vi "Startup_proximity.vi"(6 "LabVIEW Web Service":refnum<class "Web Service.lvclass">) -> ()   [LabVIEW 2019]
uses:
  <vilib>/wsapi/Web Service.lvclass
  <vilib>/httpClient/POSTBuffer.vi
  <vilib>/httpClient/LabVIEWHTTPClient.lvlib
panel:
  out "Publish Response":string[](array[string])
  # "Use the web service input terminal to call the VIs on the Service subpalette of the Web Services palette. Do not remove it from the connector pane unless you don't need access to the palette."
  # "Any additional terminals added to the connector pane of a startup VI will be ignored."
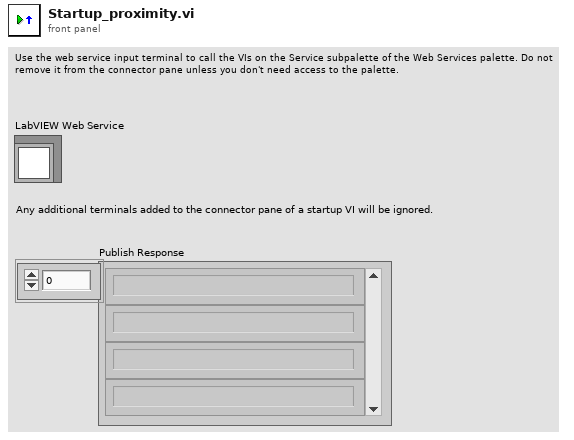
[diagram p1: front panel]
types:
  T1 = cluster{"name":string, "value":dbl[], "source":string}
  T2 = cluster{"name":string, "value":dbl[], "source":string}[]
  T3 = typedef "LabVIEWHTTPClient.lvlib/ClientHandle.ctl" = refnum<k1>
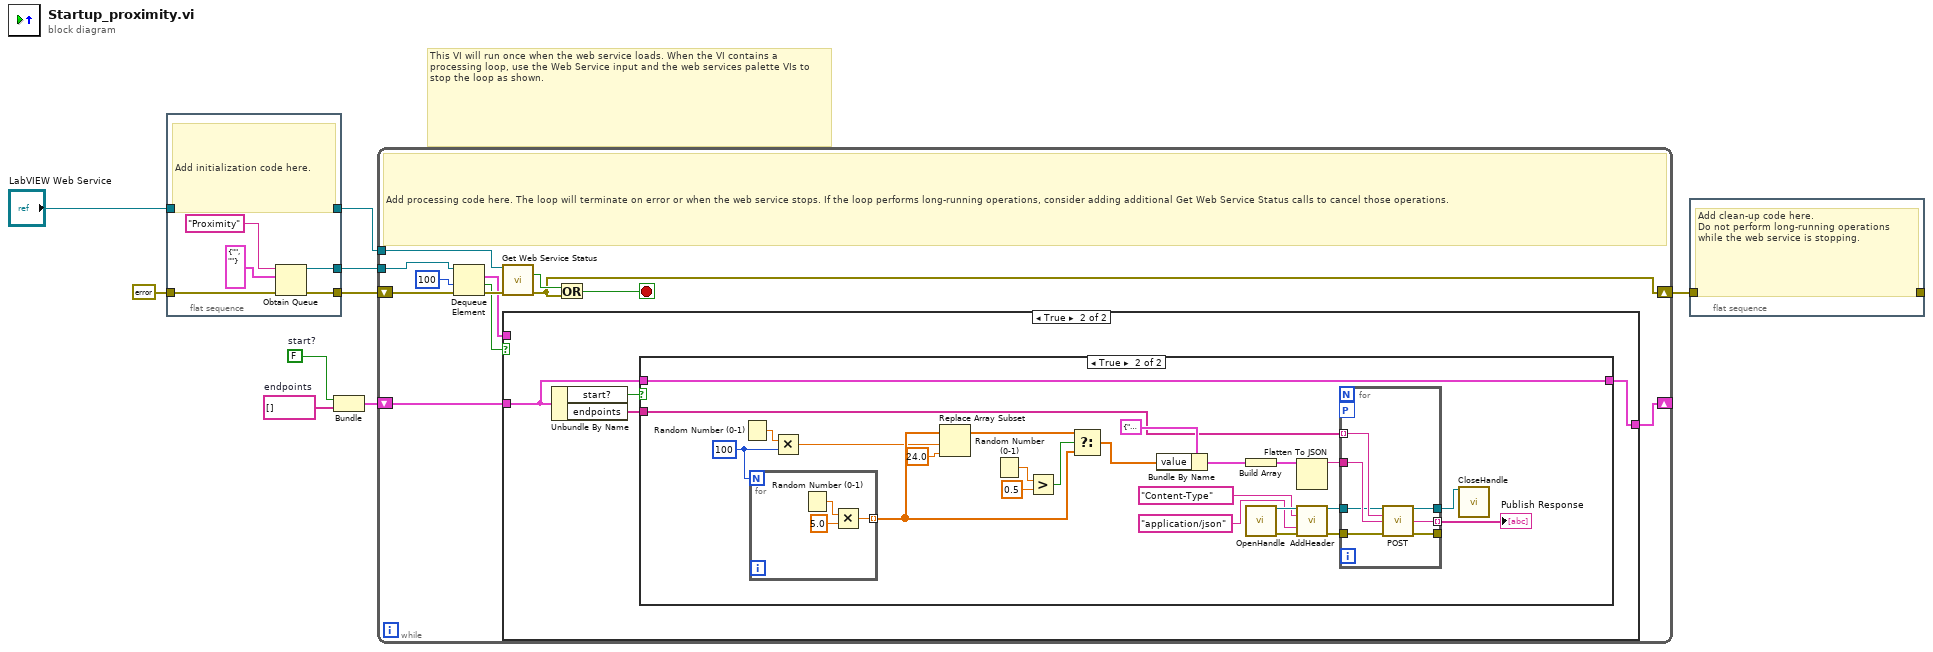
[diagram p0: block diagram]
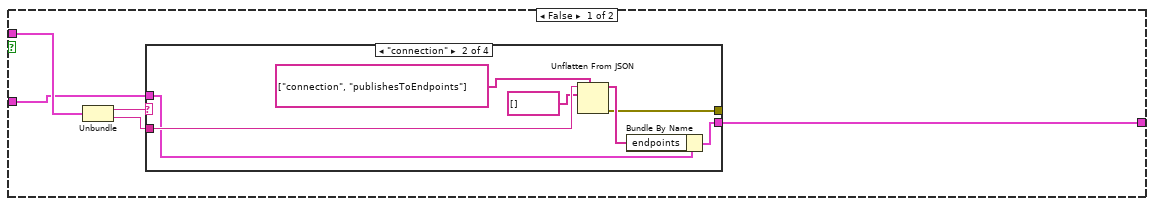
[diagram p2: hidden frame]
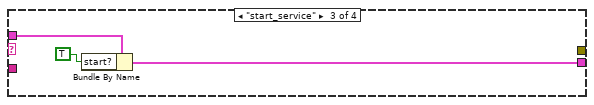
[diagram p4: hidden frame]
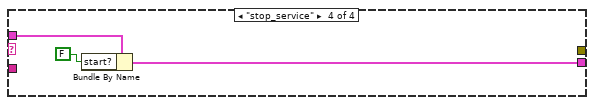
[diagram p5: hidden frame]
diagram:
  w1 = string[] []  # endpoints
  w3 = FALSE  # start?
  # "This VI will run once when the web service loads. When the VI contains a processing loop, use the Web Service input and the web services palette VIs to stop the loop as shown."
  n1 = flat-sequence {
    tunnel: "LabVIEW Web Service" -> [w15]
    tunnel: [w15] -> w8
    tunnel: [w11] -> w7
    tunnel: errorcluster {"status"=FALSE, "code"=0, "source"=""} ("error constant") -> [w10]
    tunnel: [w12] -> w4
    frame #0 {
      # "Add initialization code here."
      n2 = Obtain Queue(name (unnamed)="Proximity", element data type=cluster{string, "postdata":string} {"", "postdata"=""} ("output cluster"), error in (no error)=w10) -> (queue out=w12:refnum<queue>, error out=w11:errorcluster)  [unwired: 2 in, 1 out]
    }
  }
  n3 = Bundle("start?"=w3, "endpoints"=w1) -> (w2:cluster{"start?":bool, "endpoints":string[]})  [unwired: 1 in]
  n4 = while {
    tunnel: w8 -> [w26]
    shift-right: [w24] -> w5
    shift-left: w7 -> [w23]
    tunnel: w4 -> [w21]
    shift-right: [w16] -> _
    shift-left: w2 -> [w18]
    stop <- w25 stop-if-true
    # "Add processing code here. The loop will terminate on error or when the web service stops. If the loop performs long-running operations, consider adding additional Get Web Service Status calls to cancel those operations."
    n5 = Dequeue Element(queue=w21, timeout in ms (-1)=100, error in (no error)=w23) -> (element=w17:cluster{string, "postdata":string}, timed out?=w19:bool, error out=w22:errorcluster)  [unwired: 1 out]
    n6 = call <vilib>:"Get Web Service Status.vi"("LabVIEW Web Service"=w26, "error in (no error)"=w22) -> ("service stopping?"=w27:bool, "error out"=w24:errorcluster)  [unwired: 11 in, 1 out]
    n7 = case shown="True" w19 {
      tunnel: w18 -> [w29 w48]
      tunnel: w17 -> [w32 _]
      tunnel: [w28 w49] -> w16
      frame False {
        n8 = Unbundle(w32) -> (w31:string, "postdata"=w30:string)
        n9 = case shown="\"connection\"" w31 {
          tunnel: w30 -> [_ w40 _ _]
          tunnel: w29 -> [w33 w37 w43 w46]
          tunnel: [_ w35 _ _] -> _
          tunnel: [w33 w34 w42 w45] -> w28
          frame Default {
          }
          frame "connection" {
            n10 = Unflatten From JSON(path=string[] ["connection", "publishesToEndpoints"], JSON string=w40, type and defaults=string[] [] ("path")) -> (value=w36:string[], error out=w35:errorcluster)  [unwired: 4 in]
            n11 = Bundle By Name(cluster=w37, "endpoints"=w36) -> (w34:cluster{"start?":bool, "endpoints":string[]})
          }
          frame "start_service" {
            n12 = Bundle By Name(cluster=w43, "start?"=TRUE) -> (w42:cluster{"start?":bool, "endpoints":string[]})
          }
          frame "stop_service" {
            n13 = Bundle By Name(cluster=w46, "start?"=FALSE) -> (w45:cluster{"start?":bool, "endpoints":string[]})
          }
        }
      }
      frame True {
        n14 = Unbundle By Name(w48) -> ("start?"=w50:bool, "endpoints"=w47:string[])
        n15 = case shown="True" w50 {
          tunnel: [w51 w75] -> w49
          tunnel: w48 -> [w51 w75]
          tunnel: w47 -> [_ w63]
          frame False {
          }
          frame True {
            w66 = 100
            n16 = Random Number (0-1)() -> (number: 0 to 1=w67:dbl)
            n17 = for {
              N: w66 -> [_]
              tunnel: [w83] -> w70 mode=indexing
              n18 = Random Number (0-1)() -> (number: 0 to 1=w85:dbl)
              n19 = Multiply(x=w85, y=5.0) -> (x*y=w83:dbl)
            }
            n20 = Multiply(x=w67, y=w66) -> (x*y=w65:dbl)
            n21 = Replace Array Subset(array=w70, new element=24.0 ("new element/subarray"), index=w65) -> (w69:dbl[])
            n22 = Random Number (0-1)() -> (number: 0 to 1=w73:dbl)
            n23 = Greater?(x=w73, y=0.5) -> (0:w72:bool)
            n24 = Select(t=w69, s=w72, f=w70) -> (s? t:f=w71:dbl[])
            n25 = Bundle By Name(cluster=T1 {"name"="Promximity Sensor", "value"=[], "source"="Promximity Sensor"}, "value"=w71) -> (w62:T1)
            n26 = Build Array(w62) -> (w61:T2)
            n27 = call <vilib>:"OpenHandle.vi"() -> ("client handle out"=w57:T3, "error out"=w56:errorcluster)  [unwired: 14 in]
            n28 = Flatten To JSON(anything=w61) -> (JSON string=w60:string)  [unwired: 2 in, 1 out]
            n29 = call <vilib>:"AddHeader.vi"("client handle"=w57, "header"="Content-Type", "value"="application/json", "error in (no error)"=w56) -> ("client handle out"=w54:T3, "error out"=w55:errorcluster)  [unwired: 10 in]
            n30 = for {
              tunnel: w63 -> [w82] mode=indexing
              tunnel: w60 -> [w81]
              tunnel: [w80] -> w59 mode=indexing
              workers-P: _ -> [_]
              tunnel: w55 -> [w77]
              tunnel: [w76] -> _
              tunnel: w54 -> [w79]
              tunnel: [w78] -> w58
              n31 = call-poly <vilib>:"POST.vi"("client handle"=w79, "url"=w82, "buffer"=w81, "error in (no error)"=w77) -> ("client handle out"=w78:T3, "body"=w80:string, "error out"=w76:errorcluster)  [unwired: 8 in, 1 out]
            }
            "Publish Response" <- w59
            n32 = call <vilib>:"CloseHandle.vi"("client handle"=w58) -> ()  [unwired: 14 in, 1 out]
          }
        }
      }
    }
    n33 = Or(x=w27, y=w24) -> (x .or. y?=w25:bool)
  }
  n34 = flat-sequence {
    tunnel: [w86] -> _
    tunnel: w5 -> [w86]
    frame #0 {
      # "Add clean-up code here.\nDo not perform long-running operations while the web service is stopping."
    }
  }
